vi "Initiate Autotune.vi"(0 "VISA resource name":refnum<visa-resource-name>, 1 "Initiate Autotune (T: Yes)":bool=TRUE, 5 "Output's Control Loop (1:1)":u16(ring)=1 items=["1"=1, "2"=2], 7 "Mode (0:P Only)":u16(ring) items=["P Only", "P and I", "P, I, and D"], 11 "error in (no error)":errorcluster) -> (4 "VISA resource name out":refnum<visa-resource-name>, 15 "error out":errorcluster)   [LabVIEW 2019, in "Lake Shore 335.lvlib"]
doc: "Initiates the Autotune process. Before initiating the Autotune process, the colling system must be configured properly with control input sensor and heater output making it capable of closed-looop cotrol. The control sensor must have a valid temperature response curve assigned to it. An appropriate heater range must also be determined. The system must be coarsely maintaining temperature within 5 k of the setpoint where new tuning parameters are desired in order for the Autotuning process to initiate."
uses:
  Lake Shore 335.lvlib
  Instance           1 25Saved   Initiate Autotune .vi
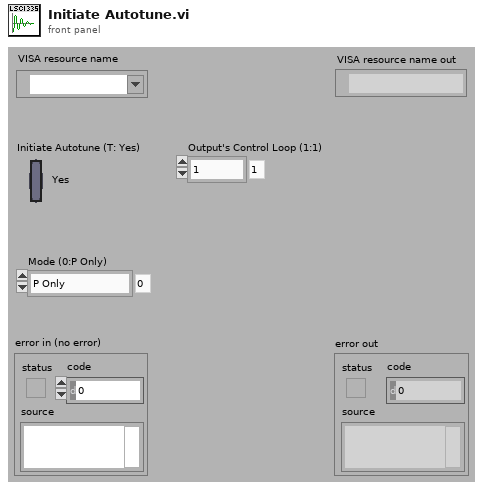
[diagram p1: front panel]
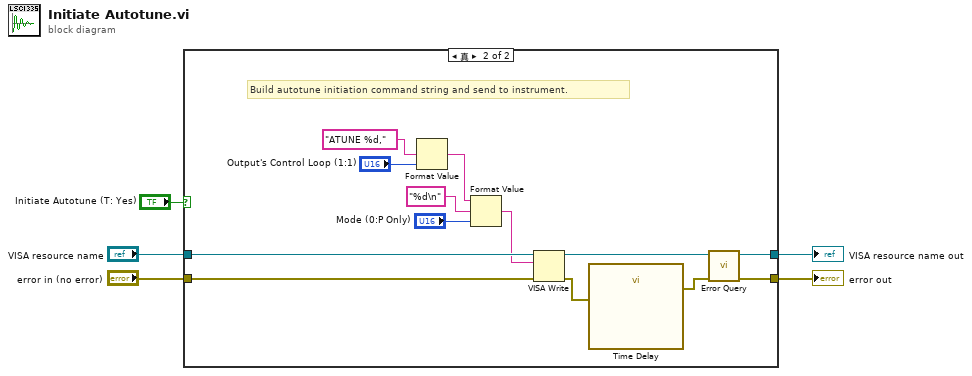
[diagram p0: block diagram]
diagram:
  n1 = case shown="真" "Initiate Autotune (T: Yes)" {
    tunnel: "VISA resource name" -> [w7 w20]
    tunnel: "error in (no error)" -> [w6 w19]
    tunnel: [w7 w17] -> w3
    tunnel: [w6 w16] -> w2
    frame False {
      # "Do not initiate Autotune"
    }
    frame True {
      # "Build autotune initiation command string and send to instrument."
      n2 = Format Value(format string="ATUNE %d,", value (0)="Output's Control Loop (1:1)") -> (output string=w8:string)  [unwired: 1 in]
      n3 = Format Value(string ("")=w8, format string="%d\n", value (0)="Mode (0:P Only)") -> (output string=w11:string)
      n4 = VISA Write(VISA resource name=w20, write buffer=w11, error in (no error)=w19) -> (VISA resource name out=w18:refnum<visa-resource-name>, error out=w14:errorcluster)  [unwired: 1 out]
      n5 = call "Time Delay"("error in (no error)"=w14) -> ("error out"=w13:errorcluster)  [unwired: 10 in]
      n6 = call "Error Query.vi"("error in (no error)"=w13, "VISA resource name"=w18) -> ("error out"=w16:errorcluster, "VISA resource name out"=w17:refnum<visa-resource-name>)  [unwired: 7 in, 1 out]
    }
  }
  "VISA resource name out" <- w3
  "error out" <- w2
